vi "TouchPanel.Driver.vi"(7 "Driver Commands":T1, 8 "New Edit Position":i32, 9 "Initial String":string, 10 "Max Length (70)":i32=70, 11 "Character":string) -> (2 "Edit Position":i32, 3 "String Out":string)   [LabVIEW 2016]
uses:
  TouchPanel.DriverCommands.ctl
panel:
  # "Inputs"
  # "Outputs"
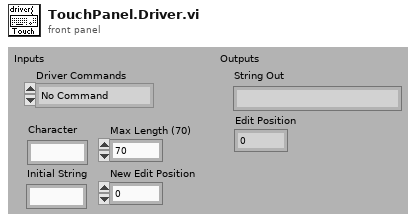
[diagram p1: front panel]
types:
  T1 = typedef "TouchPanel.DriverCommands.ctl" = enum16{"No Command", "Initialize", "Add Character", "Replace Character", "Delete Character", "Move Left", "Move Right", "Update Edit Position"}
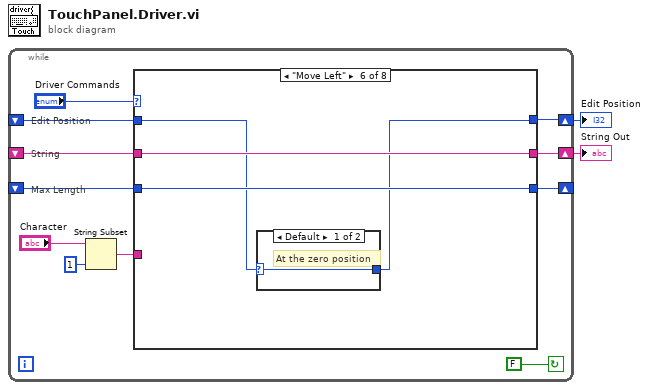
[diagram p0: block diagram]
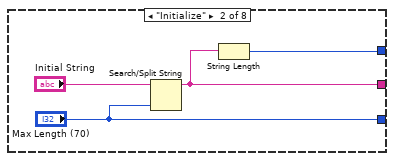
[diagram p3: hidden frame]
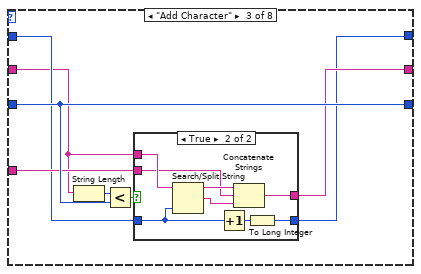
[diagram p4: hidden frame]
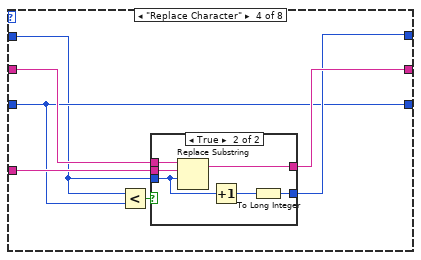
[diagram p6: hidden frame]
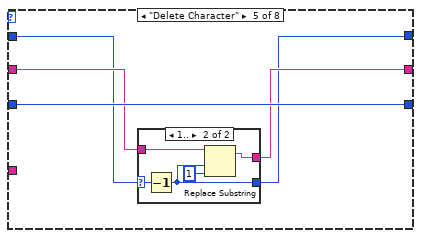
[diagram p8: hidden frame]
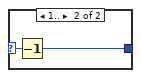
[diagram p10: hidden frame]
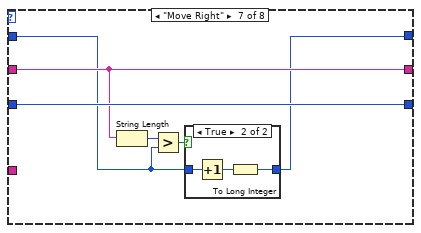
[diagram p11: hidden frame]
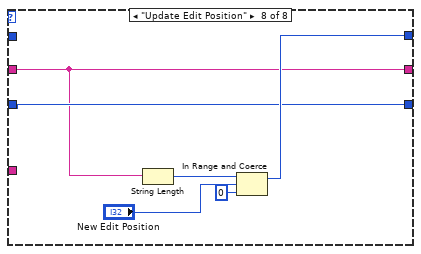
[diagram p13: hidden frame]
diagram:
  n1 = while {
    shift-right: [w11] -> w1
    shift-left: _ -> [w10]
    shift-right: [w12] -> w2
    shift-left: _ -> [w9]
    shift-right: [w7] -> _
    shift-left: _ -> [w6]
    stop <- FALSE continue-if-true
    # "Max Length"
    # "String"
    # "Edit Position"
    n2 = String Subset(string="Character", length (rest)=1 ("length (rest)")) -> (substring=w3:string)  [unwired: 1 out]
    n3 = case shown="\"Move Left\"" "Driver Commands" {
      tunnel: [w15 w19 w24 w44 w57 w69 w75 w84] -> w12
      tunnel: [w16 w20 w22 w43 w54 w66 w73 w86] -> w11
      tunnel: w10 -> [w16 _ w23 w39 w55 w67 w74 _]
      tunnel: w9 -> [w15 _ w21 w42 w56 w69 w75 w84]
      tunnel: [w14 "Max Length (70)" w27 w41 w58 w68 w78 w85] -> w7
      tunnel: w6 -> [w14 _ w27 w41 w58 w68 w78 w85]
      tunnel: w3 -> [_ _ w26 w45 _ _ _ _]
      frame "No Command" {
      }
      frame "Initialize" {
        n4 = Search/Split String(string="Initial String", offset (0)="Max Length (70)") -> (substring before match=w19:string)  [unwired: 3 out]
        n5 = String Length(string=w19) -> (length=w20:i32)
      }
      frame "Add Character" {
        n6 = String Length(string=w21) -> (length=w28:i32)
        n7 = Less?(x=w28, y=w27) -> (x < y?=w25:bool)
        n8 = case shown="True" w25 {
          tunnel: w26 -> [_ w31]
          tunnel: w23 -> [w29 w36]
          tunnel: [w30 w35] -> w24
          tunnel: [w29 w33] -> w22
          tunnel: w21 -> [w30 w32]
          frame False {
          }
          frame True {
            n9 = Search/Split String(string=w32, offset (0)=w36) -> (substring before match=w38:string, match + rest of string=w37:string)  [unwired: 2 out]
            n10 = Increment(x=w36) -> (x+1=w34:i32)
            n11 = Concatenate Strings(w38, w31, w37) -> (w35:string)
            n12 = To Long Integer(number=w34) -> (32bit integer=w33:i32)
          }
        }
      }
      frame "Replace Character" {
        n13 = Less?(x=w39, y=w41) -> (x < y?=w40:bool)
        n14 = case shown="True" w40 {
          tunnel: w42 -> [w47 w53]
          tunnel: w45 -> [_ w52]
          tunnel: [w47 w51] -> w44
          tunnel: w39 -> [w46 w48]
          tunnel: [w46 w49] -> w43
          frame False {
          }
          frame True {
            n15 = Replace Substring(3:w48, 4:w52, 5:w53) -> (1:w51:string)  [unwired: 2 out]
            n16 = Increment(x=w48) -> (x+1=w50:i32)
            n17 = To Long Integer(number=w50) -> (32bit integer=w49:i32)
          }
        }
      }
      frame "Delete Character" {
        n18 = case shown="1.." w55 {
          selector: w55 -> [w59 w62]
          tunnel: w56 -> [w60 w65]
          tunnel: [w60 w64] -> w57
          tunnel: [w59 w61] -> w54
          frame Default {
            # "At the zero position"
          }
          frame 1.. {
            n19 = Decrement(x=w62) -> (x-1=w61:i32)
            n20 = Replace Substring(2:1 ("length (len. of substring)"), 3:w61, 5:w65) -> (1:w64:string)  [unwired: 2 out]
          }
        }
      }
      frame "Move Left" {
        n21 = case shown="Default" w67 {
          selector: w67 -> [w70 w72]
          tunnel: [w70 w71] -> w66
          frame Default {
            # "At the zero position"
          }
          frame 1.. {
            n22 = Decrement(x=w72) -> (x-1=w71:i32)
          }
        }
      }
      frame "Move Right" {
        n23 = String Length(string=w75) -> (length=w76:i32)
        n24 = Greater?(x=w76, y=w74) -> (0:w77:bool)
        n25 = case shown="True" w77 {
          tunnel: w74 -> [w79 w82]
          tunnel: [w79 w80] -> w73
          frame False {
            # "At the far right"
          }
          frame True {
            n26 = Increment(x=w82) -> (x+1=w81:i32)
            n27 = To Long Integer(number=w81) -> (32bit integer=w80:i32)
          }
        }
      }
      frame "Update Edit Position" {
        n28 = String Length(string=w84) -> (length=w87:i32)
        n29 = In Range and Coerce(upper limit=w87, x="New Edit Position", lower limit=0) -> (coerced(x)=w86:i32)  [unwired: 1 out]
      }
    }
  }
  "String Out" <- w2
  "Edit Position" <- w1
